vi "Enable Relative Measurement.vi"(7 "Measurement Function (0: Current)":i32(ring) items=["Current", "Voltage", "Resistance", "Power"], 8 "error in (no error)":errorcluster, 9 "Enable Relative Measurement (F: Disable)":bool, 10 "Source Measure Unit Channel (0: Channel A)":i32(ring) items=["Channel A", "Channel B"], 11 "VISA resource name":refnum<visa-resource-name>) -> (0 "error out":errorcluster, 3 "VISA resource name out":refnum<visa-resource-name>)   [LabVIEW 2017, in "Keithley 2600 Series.lvlib"]
doc: "Enables or disables the relative measurements. \n\n<b>Note:</b>\nWhen relative measurements are enabled, all subsequent measured readings will be offset by the relative offset value specified by <b>Configure Relative Measurement Level </b>VI."
uses:
  <instrlib>/Keithley 2600 Series/Keithley 2600 Series.lvlib
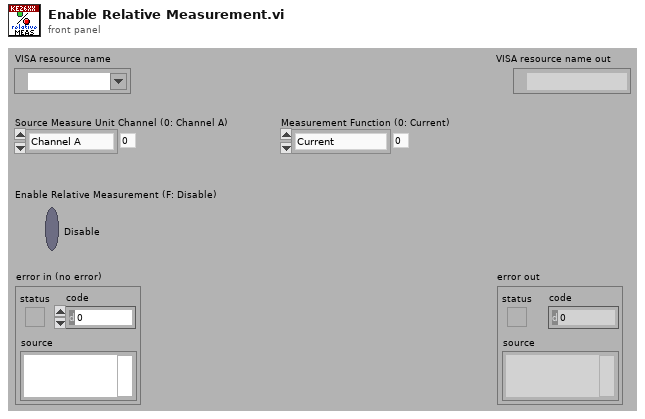
[diagram p1: front panel]
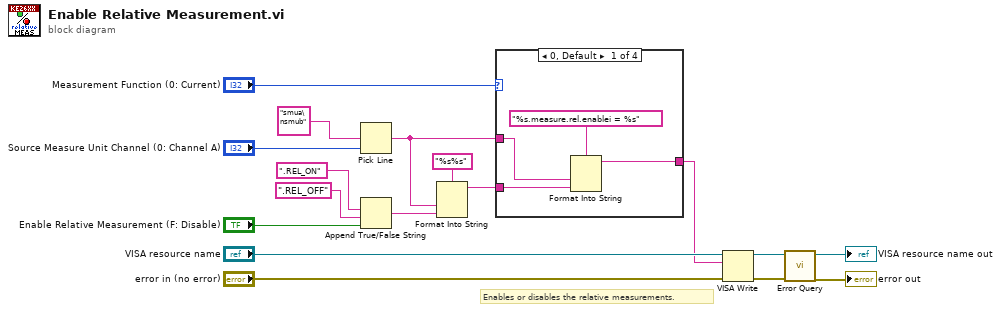
[diagram p0: block diagram]
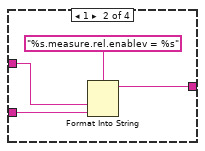
[diagram p2: hidden frame]
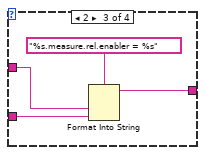
[diagram p3: hidden frame]
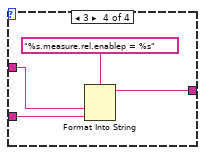
[diagram p4: hidden frame]
diagram:
  # "Enables or disables the relative measurements."
  n1 = Pick Line(multi-line string="smua\nsmub", line index="Source Measure Unit Channel (0: Channel A)") -> (output string=w2:string)  [unwired: 1 in]
  n2 = Append True/False String(1:"Enable Relative Measurement (F: Disable)", 2:".REL_OFF", 3:".REL_ON") -> (0:w5:string)  [unwired: 1 in]
  n3 = Format Into String(format string="%s%s", w2, w5) -> (resulting string=w4:string)  [unwired: 2 in, 1 out]
  n4 = case shown="0, Default" "Measurement Function (0: Current)" {
    tunnel: w4 -> [w20 w24 w28 w31]
    tunnel: w2 -> [w19 w23 w27 w30]
    tunnel: [w18 w22 w26 w32] -> w1
    frame 0, Default {
      n5 = Format Into String(format string="%s.measure.rel.enablei = %s", w19, w20) -> (resulting string=w18:string)  [unwired: 2 in, 1 out]
    }
    frame 1 {
      n6 = Format Into String(format string="%s.measure.rel.enablev = %s", w23, w24) -> (resulting string=w22:string)  [unwired: 2 in, 1 out]
    }
    frame 2 {
      n7 = Format Into String(format string="%s.measure.rel.enabler = %s", w27, w28) -> (resulting string=w26:string)  [unwired: 2 in, 1 out]
    }
    frame 3 {
      n8 = Format Into String(format string="%s.measure.rel.enablep = %s", w30, w31) -> (resulting string=w32:string)  [unwired: 2 in, 1 out]
    }
  }
  n9 = VISA Write(VISA resource name="VISA resource name", write buffer=w1, error in (no error)="error in (no error)") -> (VISA resource name out=w12:refnum<visa-resource-name>, error out=w11:errorcluster)  [unwired: 1 out]
  n10 = call <instrlib>:"Error Query.vi"("error in (no error)"=w11, "VISA resource name"=w12) -> ("error out"=→"error out":errorcluster, "VISA resource name out"=→"VISA resource name out":refnum<visa-resource-name>)  [unwired: 6 in, 2 out]
